vi "Read last phase.vi"(8 "error in (no error)":errorcluster, 11 "ScopeBase in":refnum<class "ScopeBase.lvclass">) -> (0 "error out":errorcluster, 2 "last phase":dbl[](array[numeric]), 3 "ScopeBase out":refnum<class "ScopeBase.lvclass">)   [LabVIEW 2013, in "ScopeBase.lvclass"]
uses:
  ScopeBase.lvclass
  ScopeBase.lvclass/ScopeBase.ctl
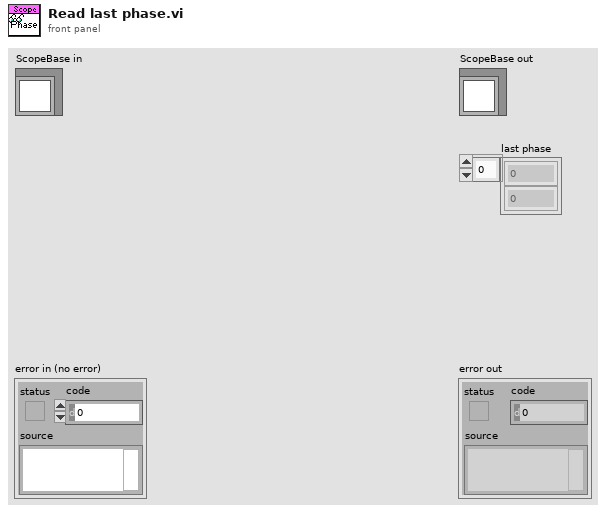
[diagram p1: front panel]
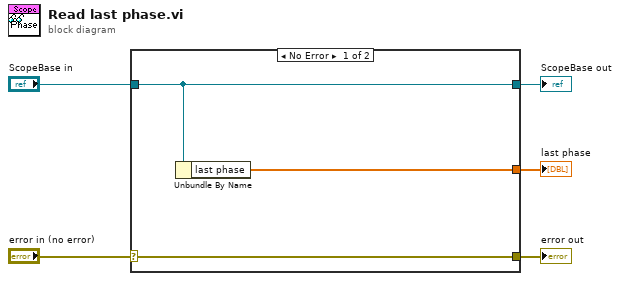
[diagram p0: block diagram]
diagram:
  n1 = case shown="No Error" "error in (no error)" {
    selector: "error in (no error)" -> [w8 w9]
    tunnel: [w8 w9] -> w4
    tunnel: [w7 w10] -> w2
    tunnel: "ScopeBase in" -> [w7 w10]
    tunnel: [w6 _] -> w1
    frame No Error {
      n2 = Unbundle By Name(w7) -> ("last phase"=w6:dbl[])
    }
    frame Error {
    }
  }
  "error out" <- w4
  "ScopeBase out" <- w2
  "last phase" <- w1
